vi "7.quick-run-for-loop.vi"() -> ()   [LabVIEW 2010]
panel:
  in  "stop":bool
  in  "# of time to  run":dbl
  out "current-iteration-no":dbl
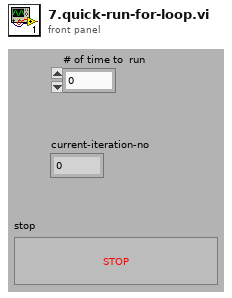
[diagram p1: front panel]
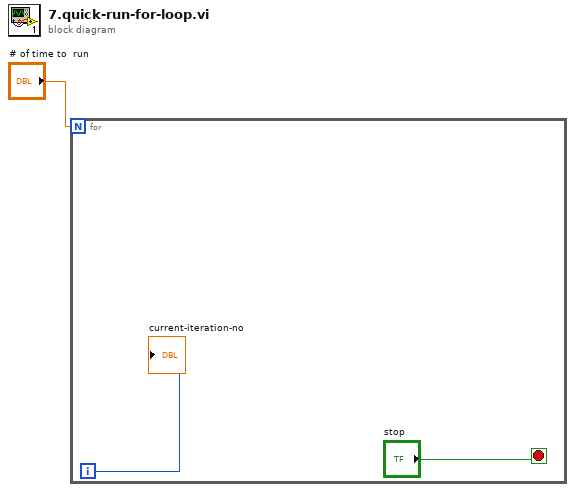
[diagram p0: block diagram]
diagram:
  n1 = for {
    N: "# of time to  run" -> [_]
    i -> [w3]
    stop <- "stop" stop-if-true
    "current-iteration-no" <- w3
  }
